vi "DrawCircle.vi"(1 "y":dbl, 2 "x":dbl, 3 "r":i32=360) -> (0 "XY Graph":cluster{dbl[], dbl[]}(graph))   [LabVIEW 2014]
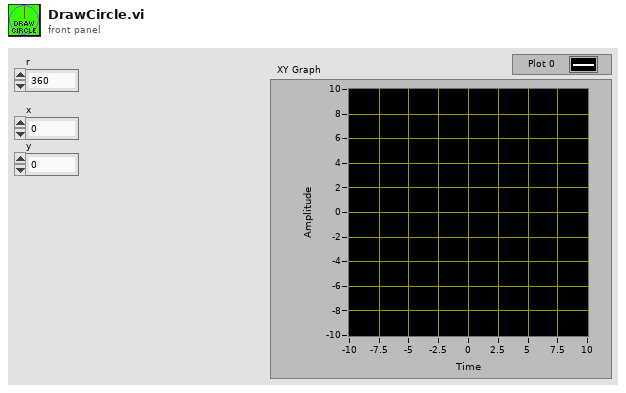
[diagram p1: front panel]
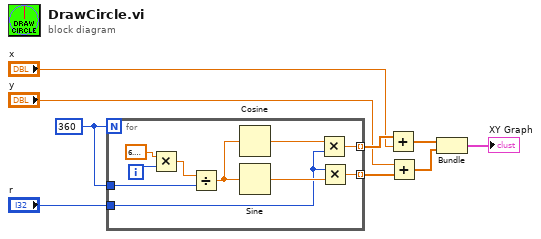
[diagram p0: block diagram]
diagram:
  w9 = 360
  n1 = for {
    N: w9 -> [_]
    tunnel: w9 -> [w16]
    tunnel: [w12] -> w8 mode=indexing
    tunnel: [w11] -> w7 mode=indexing
    tunnel: "r" -> [w10]
    i -> [w18]
    n2 = Multiply(x=6.283185307179586, y=w18) -> (x*y=w17:dbl)
    n3 = Divide(x=w17, y=w16) -> (x/y=w15:dbl)
    n4 = Cosine(x=w15) -> (cos(x)=w14:dbl)
    n5 = Sine(x=w15) -> (sin(x)=w13:dbl)
    n6 = Multiply(x=w14, y=w10) -> (x*y=w12:dbl)
    n7 = Multiply(x=w10, y=w13) -> (x*y=w11:dbl)
  }
  n8 = Add(x=w8, y="x") -> (x+y=w4:dbl[])
  n9 = Add(x="y", y=w7) -> (x+y=w3:dbl[])
  n10 = Bundle(w4, w3) -> (→"XY Graph":cluster{dbl[], dbl[]})  [unwired: 1 in]
